vi "Load Plugin.vi"(6 "Version String":string, 7 "Directory":path=path "/home/lvuser/natinst/bin", 8 "error in (no error)":errorcluster, 9 "Unique Name":string, 10 "Plugin Type":string="CIFTemplatePlugin", 11 "Launcher in":refnum<class "Plugin Manager.lvclass">) -> (0 "error out":errorcluster, 3 "Launcher out":refnum<class "Plugin Manager.lvclass">)   [LabVIEW 2021, in "Plugin Manager.lvclass"]
uses:
  Plugin Manager.lvclass
  Plugin Manager.lvclass/Plugin Manager.ctl
  CIFCore/Common/Typedef/Errors.ctl
  typedef/Plugin Management Data.ctl
  CIFCore/Common/Typedef/Version.ctl
  CIFCore/Common/Utilities/Append Error Location.vi
  CIFUtilities/CIFClocks/Time Conversion/LabVIEW Time to UTC Time.vi
  <vilib>/Utility/LVLibp/NI_PackedLibraryUtility.lvlib
  CIFCore/Common/CIFCoreCommon.lvlib
  CIFUtilities/CIFClocks/CIFClocks.lvlib
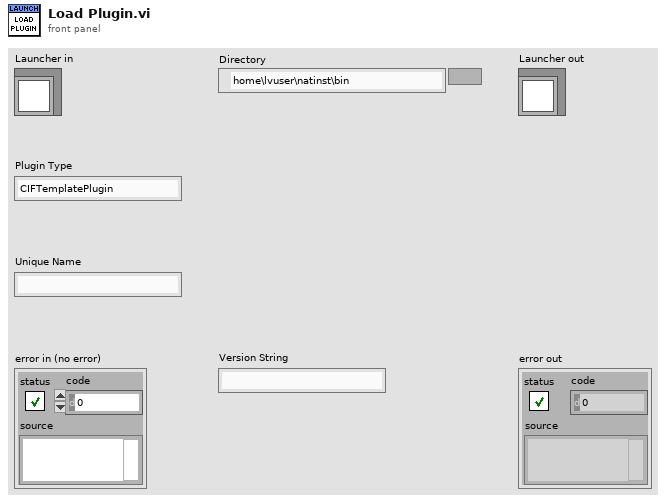
[diagram p1: front panel]
types:
  T1 = typedef "CIFCoreCommon.lvlib/Errors.ctl" = enum16{"Invalid Clock ID", "Long Sleep", "gRPC Server Not Found", "Config Parse", "Timestamp Wrap", "Delayed Execution", "Duplicate Channel", "Missing Channel", "Incorrect Type", "Flatten Error", "Unflatten Data", "Unique Name", "Plugin Not Found"}
  T2 = typedef "Plugin Manager.lvclass/Plugin Management Data.ctl" = cluster{"vi reference":refnum<vi>, "Plugin Type":string, "Unique Name":string, "Load Timestamp":u64, "gRPC Port":i32, "Version":T3}
  T3 = typedef "CIFCoreCommon.lvlib/Version.ctl" = cluster{"Major":i32, "Minor":i32, "Fix":i32, "Build":i32}
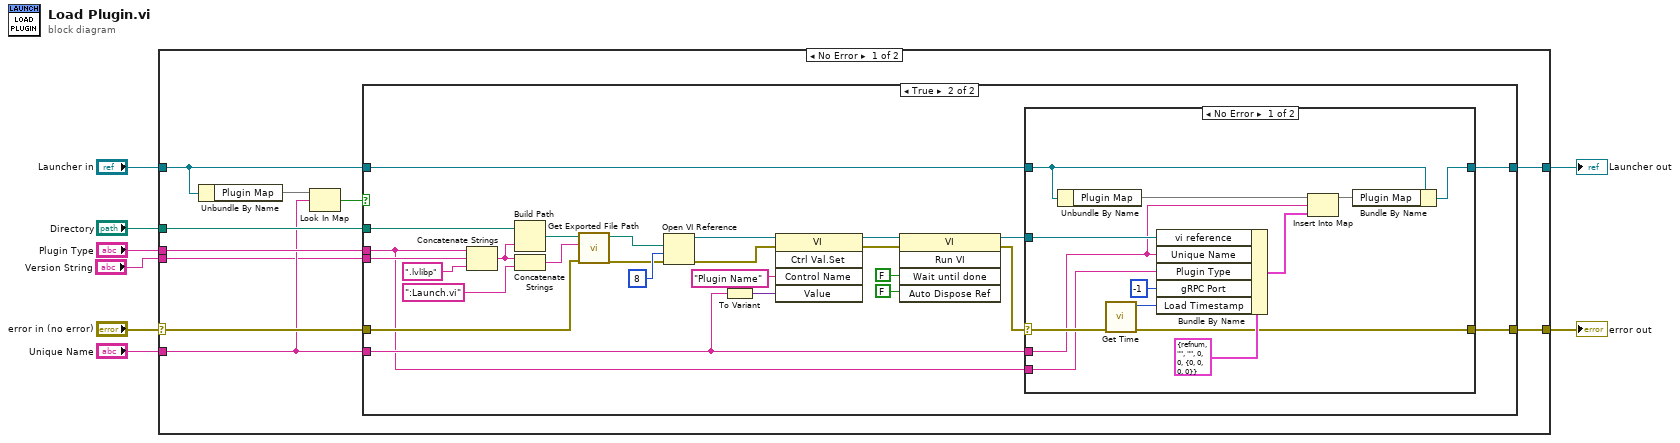
[diagram p0: block diagram]
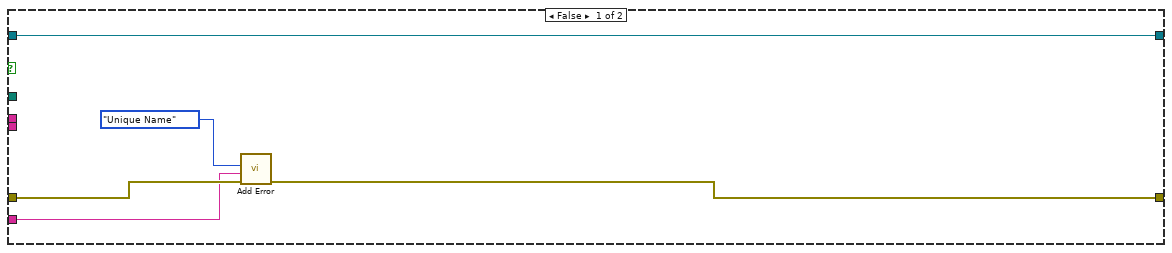
[diagram p2: hidden frame]
diagram:
  n1 = case shown="No Error" "error in (no error)" {
    selector: "error in (no error)" -> [w17 w66]
    tunnel: [w16 w66] -> w7
    tunnel: [w12 w65] -> w5
    tunnel: "Launcher in" -> [w9 w65]
    tunnel: "Directory" -> [w18 _]
    tunnel: "Plugin Type" -> [w15 _]
    tunnel: "Unique Name" -> [w14 _]
    tunnel: "Version String" -> [w10 _]
    frame No Error {
      n2 = Unbundle By Name(w9) -> ("Plugin Map"=w13:map{string, T2})
      n3 = Look In Map(map=w13, key=w14) -> (key not found?=w11:bool)  [unwired: 1 in, 1 out]
      n4 = case shown="True" w11 {
        tunnel: w18 -> [_ w47]
        tunnel: w17 -> [w23 w46]
        tunnel: [w20 w26] -> w16
        tunnel: w15 -> [_ w25]
        tunnel: w14 -> [w21 w28]
        tunnel: w9 -> [w19 w27]
        tunnel: [w19 w24] -> w12
        tunnel: w10 -> [_ w32]
        frame False {
          n5 = call "Add Error.vi"("error in (no error)"=w23, "String to Append"=w21, "Error"=Errors."Unique Name") -> ("error out"=w20:errorcluster)  [unwired: 8 in]
        }
        frame True {
          n6 = Concatenate Strings(w25, w32, ".lvlibp" ("string")) -> (w33:string)
          n7 = Build Path(base path=w47, name or relative path=w33) -> (appended path=w48:path)
          n8 = Concatenate Strings(w33, ":Launch.vi" ("qualified name")) -> (w34:string)
          n9 = call <vilib>:"Get Exported File Path.vi"("error in (no error)"=w46, "qualified name"=w34, "packed library path"=w48) -> ("error out"=w37:errorcluster, "path"=w38:path)  [unwired: 7 in]
          n10 = Open VI Reference(vi path=w38, options=8, error in (no error)=w37) -> (vi reference=w40:refnum<vi>, error out=w43:errorcluster)  [unwired: 3 in]
          n11 = To Variant(anything=w28) -> (Variant=w36:variant)
          n12 = invoke class="VI" method="Ctrl Val.Set"(reference=w40, error in=w43, "Control Name"="Plugin Name", "Value"=w36) -> (reference out=w42:refnum<vi>, error out=w41:errorcluster)  [unwired: 1 in, 3 out]
          n13 = invoke class="VI" method="Run VI"(reference=w42, error in=w41, "Wait until done"=FALSE ("Wait Until Done"), "Auto Dispose Ref"=FALSE ("Auto Dispose Reference")) -> (reference out=w29:refnum<vi>, error out=w30:errorcluster)  [unwired: 1 in, 3 out]
          n14 = case shown="No Error" w30 {
            selector: w30 -> [w60 w63]
            tunnel: w29 -> [w62 _]
            tunnel: w28 -> [w56 _]
            tunnel: w27 -> [w54 w64]
            tunnel: [w59 w63] -> w26
            tunnel: w25 -> [w58 _]
            tunnel: [w52 w64] -> w24
            frame No Error {
              n15 = Unbundle By Name(w54) -> ("Plugin Map"=w57:map{string, T2})
              n16 = call "Get Time.vi"("error in (no error)"=w60) -> ("error out"=w59:errorcluster, "Time (ns)"=w51:u64)  [unwired: 8 in, 1 out]
              n17 = Bundle By Name(cluster=T2 {"vi reference"=refnum, "Plugin Type"="", "Unique Name"="", "Load Timestamp"=0, "gRPC Port"=0, "Version"={"Major"=0, "Minor"=0, "Fix"=0, "Build"=0}} ("Plugin Management Data"), "vi reference"=w62, "Unique Name"=w56, "Plugin Type"=w58, "gRPC Port"=-1, "Load Timestamp"=w51) -> (w55:T2)
              n18 = Insert Into Map(map in=w57, key=w56, value=w55) -> (map out=w53:map{string, T2})  [unwired: 2 out]
              n19 = Bundle By Name(cluster=w54, "Plugin Map"=w53) -> (w52:refnum<class "Plugin Manager.lvclass">)
            }
            frame Error {
            }
          }
        }
      }
    }
    frame Error {
    }
  }
  "error out" <- w7
  "Launcher out" <- w5
